vi "motor speaker.vi"(10 "Vertical Pointer Slide":dbl) -> ()   [LabVIEW 2019]
uses:
  motor enum.ctl
panel:
  in  "Enum":T1
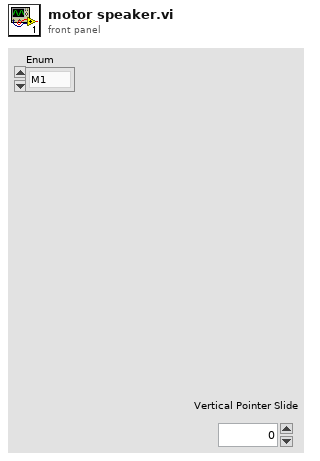
[diagram p1: front panel]
types:
  T1 = typedef "motor enum.ctl" = enum16{"M1", "M2", "M3", "M4"}
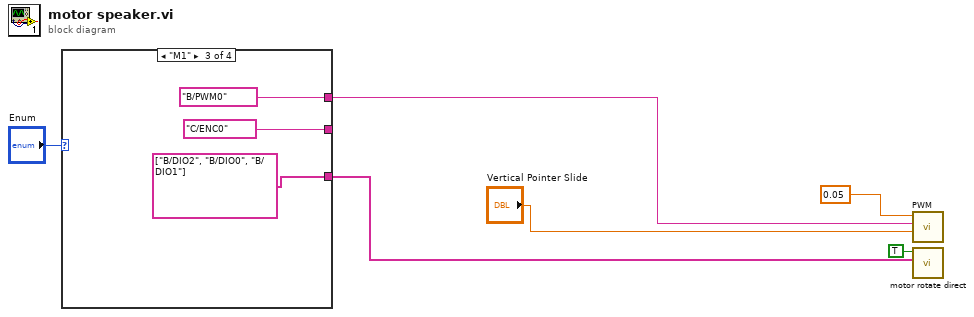
[diagram p0: block diagram]
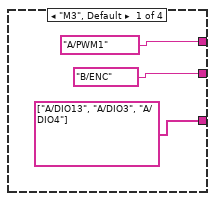
[diagram p2: hidden frame]
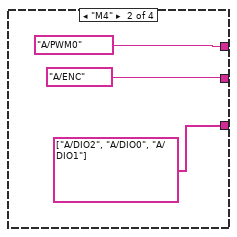
[diagram p3: hidden frame]
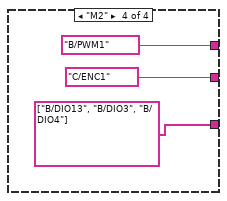
[diagram p4: hidden frame]
diagram:
  n1 = case shown="\"M1\"" "Enum" {
    tunnel: [tag "B/ENC" ("Channel Name") tag "A/ENC" ("Channel Name") tag "C/ENC0" ("Channel Name") tag "C/ENC1" ("Channel Name")] -> _
    tunnel: [tag[] ["A/DIO13", "A/DIO3", "A/DIO4"] ("Channel Names") tag[] ["A/DIO2", "A/DIO0", "A/DIO1"] ("Channel Names") tag[] ["B/DIO2", "B/DIO0", "B/DIO1"] ("Channel Names") tag[] ["B/DIO13", "B/DIO3", "B/DIO4"] ("Channel Names")] -> w5
    tunnel: [tag "A/PWM1" ("Channel Name") tag "A/PWM0" ("Channel Name") tag "B/PWM0" ("Channel Name") tag "B/PWM1" ("Channel Name")] -> w4
    frame "M3", Default {
    }
    frame "M4" {
    }
    frame "M1" {
    }
    frame "M2" {
    }
  }
  n2 = call "PWM.vi"("Frequency [Hz]"="Vertical Pointer Slide", "Channel Name"=w4, "Duty Cycle"=0.05) -> ()  [unwired: 8 in, 1 out]
  n3 = call "motor rotate direct.vi"("Channel Names"=w5, "Boolean"=TRUE) -> ()  [unwired: 9 in, 1 out]
